vi "parseInputData.vi"(11 "String":string) -> (2 "CallsData":string[](array[string]), 3 "BoardsData":string[](array[string]))   [LabVIEW 2017]
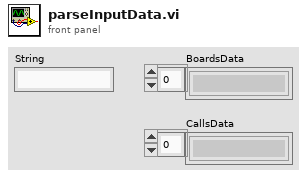
[diagram p1: front panel]
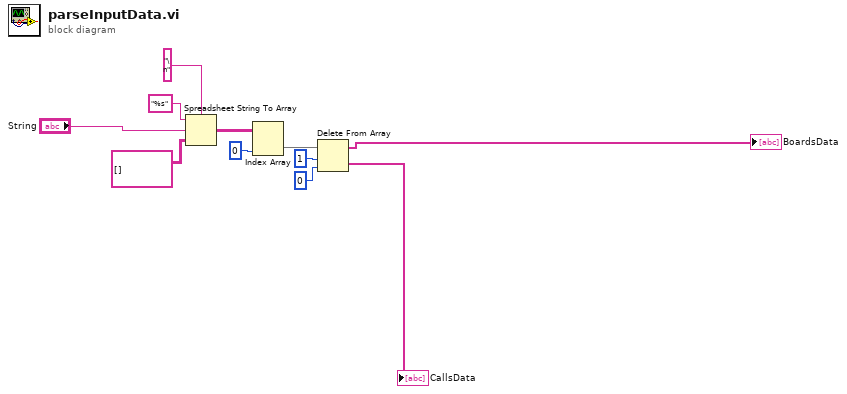
[diagram p0: block diagram]
diagram:
  n1 = Spreadsheet String To Array(delimiter (Tab)="\n", format string="%s", spreadsheet string="String", array type (2D Dbl)=string[][] []) -> (array=w7:string[][])
  n2 = Index Array(array=w7, index (col)=0 ("disabled index (col)")) -> (element=w9:string[])  [unwired: 1 in]
  n3 = Delete From Array(array=w9, length=1, index=0 ("index (row)")) -> (deleted portion=→"CallsData":string[], array with subset deleted=→"BoardsData":string[])
